vi "Database.Sets.Read.vi"(8 "error in":errorcluster) -> (0 "error out":errorcluster)   [LabVIEW 2016]
uses:
  Tools/Tma.lib/nlconfig.llb/fp2ini mode.ctl
  Global/ApplicationGlobal.vi
  Database.Global.vi
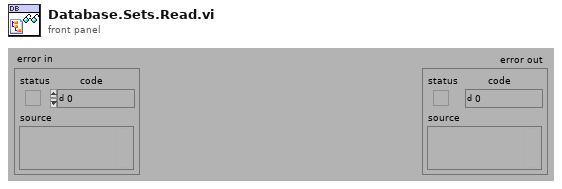
[diagram p1: front panel]
types:
  T1 = typedef "fp2ini mode.ctl" = enum16{"Read Controls", "Write Controls", "Write Indicators", "Read Indicators", "Write all", "Read all"}
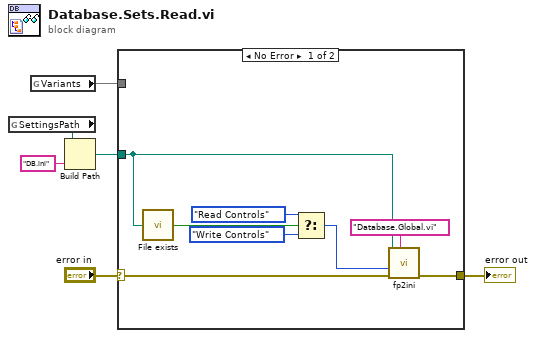
[diagram p0: block diagram]
diagram:
  n1 = global read "ApplicationGlobal.vi" "SettingsPath"() -> (w2:path)
  n2 = global read "Database.Global.vi" "Variants"() -> (w1)
  n3 = Build Path(base path=w2, name or relative path="DB.ini") -> (appended path=w3:path)
  n4 = case shown="No Error" "error in" {
    selector: "error in" -> [w13 w15]
    tunnel: [w14 w15] -> w6
    tunnel: w3 -> [w7 _]
    tunnel: w1 -> [_ _]
    frame No Error {
      n5 = call "File exists.vi"("file path"=w7) -> ("exists?"=w11:bool)  [unwired: 4 in]
      n6 = Select(t=fp2ini_mode."Read Controls" ("mode"), s=w11, f=fp2ini_mode."Write Controls" ("mode")) -> (s? t:f=w8:T1)
      n7 = call "fp2ini.vi"("vi-name (caller if empty)"="Database.Global.vi", "error in"=w13, "mode"=w8, "ini-file path"=w7) -> ("error out"=w14:errorcluster)  [unwired: 3 in, 4 out]
    }
    frame Error {
    }
  }
  "error out" <- w6
